vi "Robot Main.vi"() -> ()   [LabVIEW 2013]
doc: "This VI imlements the framework and scheduler for your robotics program. It should not be necessary to modify the framework. You are expected to add your code to the VIs called from Robot Main, the ones located in the Team Code within the project."
panel:
  in  "Finish":bool
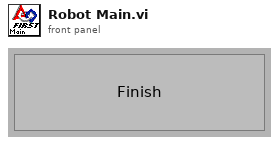
[diagram p1: front panel]
types:
  T1 = typedef "WPI_DriverStationDerivedRobotMode.ctl" = enum16{"Init", "Execute", "Stop"}
  T2 = typedef "WPI_DriverStationRobotMode.ctl" = enum16{"Autonomous Disabled", "Autonomous Enabled", "Teleop Disabled", "Teleop Enabled", "Timeout", "Finish"}
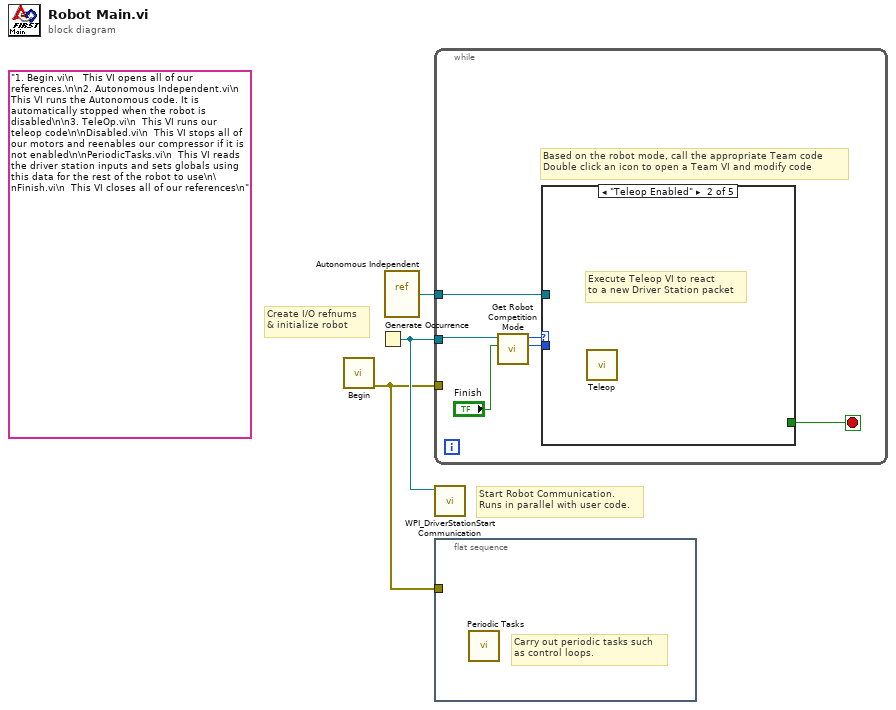
[diagram p0: block diagram]
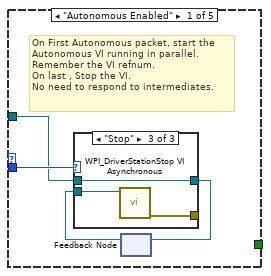
[diagram p2: hidden frame]
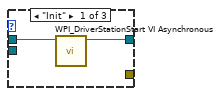
[diagram p3: hidden frame]
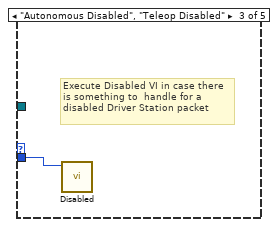
[diagram p5: hidden frame]
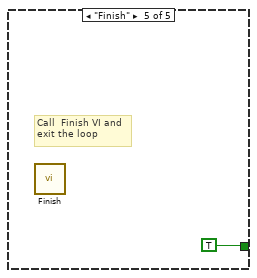
[diagram p7: hidden frame]
diagram:
  (unwired) "1. Begin.vi\n   This VI opens all of our references.\n\n2. Autonomous Independent.vi\n  This VI runs the Autonomous code. It is automatically stopped when the robot is disabled\n\n3. TeleOp.vi\n  This VI runs our teleop code\n\nDisabled.vi\n  This VI stops all of our motors and reenables our compressor if it is not enabled\n\nPeriodicTasks.vi\n  This VI reads the driver station inputs and sets globals using this data for the rest of the robot to use\n\nFinish.vi\n  This VI closes all of our references\n"
  # "Create I/O refnums\n& initialize robot"
  # "Start Robot Communication.\nRuns in parallel with user code."
  n1 = call "Begin.vi"() -> ("error out"=w2:errorcluster)  [unwired: 1 in, 10 out]
  n2 = Generate Occurrence() -> (w3:refnum<k4>)
  n3 = vi-ref "Autonomous Independent.vi"() -> (w1:refnum<vi>)
  n4 = while {
    tunnel: w3 -> [w7]
    tunnel: w2 -> [_]
    tunnel: w1 -> [w4]
    stop <- w5 stop-if-true
    # "Based on the robot mode, call the appropriate Team code\nDouble click an icon to open a Team VI and modify code"
    n5 = call "Get Robot Competition Mode.vi"("Finish"="Finish", "DS Occurrence"=w7) -> ("Call Context"=w9:T1, "Robot Mode"=w8:T2)  [unwired: 8 out]
    n6 = case shown="\"Teleop Enabled\"" w8 {
      tunnel: w9 -> [w13 _ w20 _ _]
      tunnel: [_ _ _ _ TRUE] -> w5
      tunnel: w4 -> [w12 _ _ _ _]
      frame "Autonomous Enabled" {
        # "On First Autonomous packet, start the\nAutonomous VI running in parallel.\nRemember the VI refnum.\nOn last , Stop the VI.\nNo need to respond to intermediates."
        n7 = feedback #1() -> (w10:refnum<vi>)  [unwired: 1 out]
        n8 = case shown="\"Stop\"" w13 {
          tunnel: w12 -> [w15 _ w18]
          tunnel: [w14 w16 w18] -> w11
          tunnel: w10 -> [_ w16 w19]
          tunnel: [_ _ w17] -> _
          frame "Init" {
            n9 = call <vilib>:"WPI_DriverStationStart VI Asynchronous.vi"("VI"=w15) -> ("VI out"=w14:refnum<vi>)  [unwired: 10 out]
          }
          frame "Execute", Default {
            # "Nothing to do"
          }
          frame "Stop" {
            n10 = call <vilib>:"WPI_DriverStationStop VI Asynchronous.vi"("VI Refnum"=w19) -> ("error out"=w17:errorcluster)  [unwired: 10 out]
          }
        }
        n11 = feedback-in #1(w11) -> ()
      }
      frame "Teleop Enabled" {
        # "Execute Teleop VI to react\nto a new Driver Station packet"
        n12 = call "Teleop.vi"() -> ()  [unwired: 3 in, 9 out]
      }
      frame "Autonomous Disabled", "Teleop Disabled" {
        # "Execute Disabled VI in case there\nis something to  handle for a\ndisabled Driver Station packet"
        n13 = call "Disabled.vi"("Call Context"=w20) -> ()  [unwired: 3 in, 8 out]
      }
      frame "Timeout" {
        # "Driver Station packet didn't arrive.\nPossibly useful for diagnostics"
      }
      frame "Finish" {
        # "Call  Finish VI and\nexit the loop"
        n14 = call "Finish.vi"() -> ()  [unwired: 1 in, 7 out]
      }
    }
  }
  n15 = call <vilib>:"WPI_DriverStationStart Communication.vi"("occurrence"=w3) -> ()  [unwired: 11 out]
  n16 = flat-sequence {
    tunnel: w2 -> [_]
    frame #0 {
      # "Carry out periodic tasks such\nas control loops."
      n17 = call "Periodic Tasks.vi"() -> ()  [unwired: 1 in, 11 out]
    }
  }
